vi "Scan CSM-VI.vi"(6 "Config Path":path, 8 "Error in":errorcluster caption="Error in (no error)", 11 "root":path) -> (0 "Error out":errorcluster)   [LabVIEW 2017, in "CSM-Helper API with lvcsm Support.lvlib"]
uses:
  CSM-Helper API with lvcsm Support.lvlib
panel:
  in  "Termiate":bool
  out "Path":path
  out "Slide":i32(slide) scale=0.0..1508.0
  out "All Files in Dir":path[](array[path])
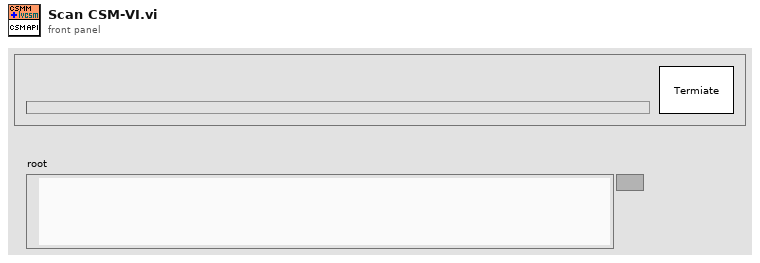
[diagram p1: front panel]
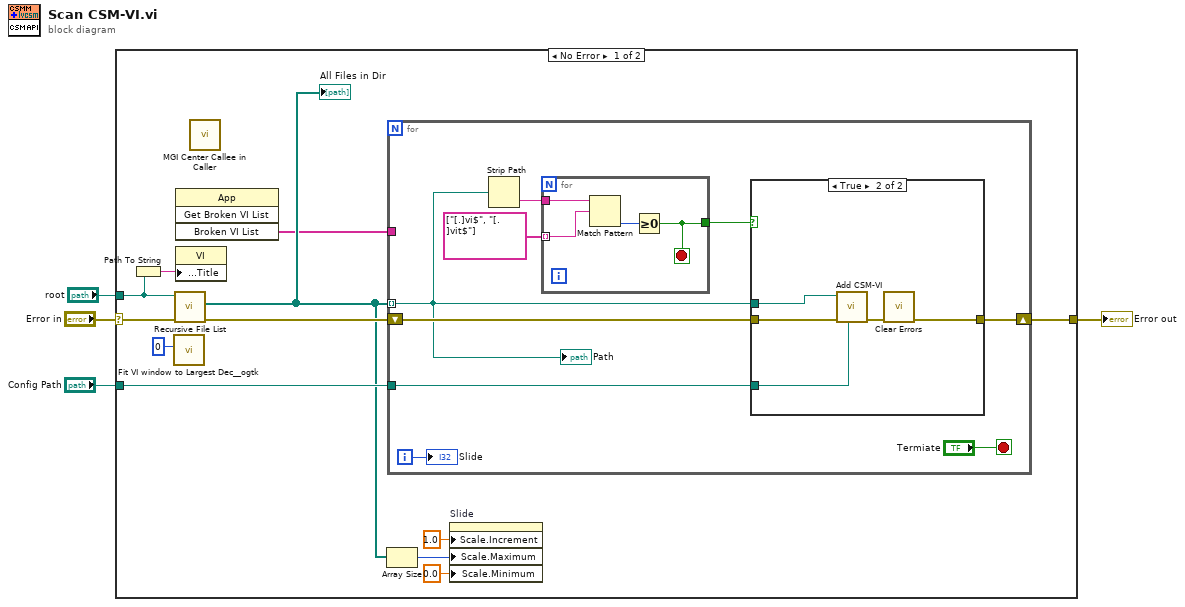
[diagram p0: block diagram]
diagram:
  n1 = case shown="No Error" "Error in" {
    selector: "Error in" -> [w16 w36]
    tunnel: [w13 w36] -> w3
    tunnel: "Config Path" -> [w15 _]
    tunnel: "root" -> [w10 _]
    frame No Error {
      n2 = Path To String(path=w10) -> (string=w11:string)
      n3 = call <userlib>:"Fit VI window to Largest Dec__ogtk.vi"("border spacing (2 px)"=0) -> ()  [unwired: 5 in, 2 out]
      n4 = call <vilib>:"Recursive File List.vi"("error in (no error)"=w16, "Folder Path"=w10) -> ("error out"=w14:errorcluster, "All Files in Dir"=w12:path[])  [unwired: 5 in, 3 out]
      "All Files in Dir" <- w12
      n5 = invoke class="App" method="Get Broken VI List"() -> ("Broken VI List"=w9:string[])  [unwired: 4 in, 3 out]
      n6 = property class="VI"("Front Panel.Title"=w11) -> ()  [unwired: 2 in, 2 out]
      n7 = call <userlib>:"MGI Center Callee in Caller.vi"() -> ()  [unwired: 11 in, 1 out]
      n8 = Array Size(array=w12) -> (size(s)=w8:i32)
      n9 = for {
        tunnel: w12 -> [w19] mode=indexing
        tunnel: w15 -> [w25]
        shift-right: [w20] -> w13
        shift-left: w14 -> [w21]
        tunnel: w9 -> [_]
        i -> [w18]
        stop <- "Termiate" stop-if-true
        n10 = Strip Path(path=w19) -> (name=w24:string)  [unwired: 1 out]
        n11 = for {
          tunnel: w24 -> [w35]
          tunnel: string[] ["[.]vi$", "[.]vit$"] ("name") -> [w34] mode=indexing
          tunnel: [w32] -> w22
          stop <- w32 stop-if-true
          n12 = Match Pattern(string=w35, regular expression=w34) -> (offset past match=w33:i32)  [unwired: 1 in, 3 out]
          n13 = Greater Or Equal To 0?(x=w33) -> (x >= 0?=w32:bool)
        }
        n14 = case shown="True" w22 {
          tunnel: w25 -> [_ w31]
          tunnel: w19 -> [_ w30]
          tunnel: w21 -> [w26 w29]
          tunnel: [w26 w27] -> w20
          frame False {
          }
          frame True {
            n15 = call "Add CSM-VI.vi"("Config Path"=w31, "error in (no error)"=w29, "CSM-VI"=w30) -> ("error out"=w28:errorcluster)  [unwired: 8 in]
            n16 = call <vilib>:"Clear Errors.vi"("error in (no error)"=w28) -> ("error out"=w27:errorcluster)  [unwired: 5 in, 1 out]
          }
        }
        "Path" <- w19
        "Slide" <- w18
      }
      n17 = property on="Slide" class="Slide (strict)"("Scale.Increment"=1.0 ("Scale.Range:Increment"), "Scale.Maximum"=w8, "Scale.Minimum"=0.0 ("Scale.Range:Minimum")) -> ()  [unwired: 2 in, 2 out]
    }
    frame Error {
    }
  }
  "Error out" <- w3
